vi "Convert Click to String.vi"(9 "Click Count":i32, 10 "Click Type":T2, 11 "Button":T1) -> (3 "Click String":string)   [LabVIEW 2020, in "MacroAssert.lvlib" / "Mouse Action.lvclass"]
uses:
  Mouse Action.lvclass
  Click Type.ctl
  Button.ctl
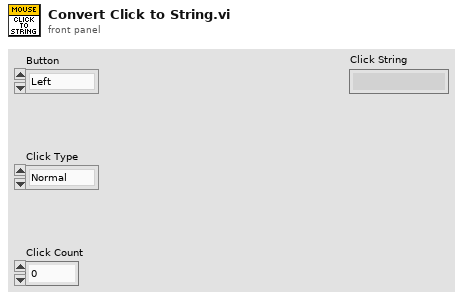
[diagram p1: front panel]
types:
  T1 = typedef "MacroAssert.lvlib/Mouse Action.lvclass/Button.ctl" = enum16{"Left", "Right", "Middle"}
  T2 = typedef "MacroAssert.lvlib/Mouse Action.lvclass/Click Type.ctl" = enum16{"Normal", "Hold", "Release"}
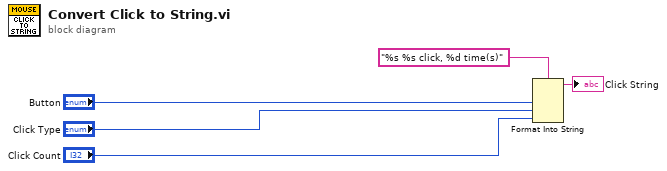
[diagram p0: block diagram]
diagram:
  n1 = Format Into String(format string="%s %s click, %d time(s)", "Button", "Click Type", "Click Count") -> (resulting string=→"Click String":string)  [unwired: 2 in, 1 out]
